vi "To Pythonic - Tuple.vi"(4 "Pythonic Values":string[](array[string])) -> (1 "Tuple":string)   [LabVIEW 2020, in "OPI.lvclass"]
doc: "Convert LabVIEW data into valid pythonic representation. \n\nThe input aray of strings should be valid pythonic values created with previous calls to To Pythonic converter."
uses:
  OPI.lvclass
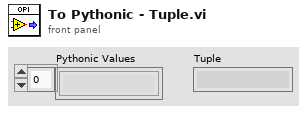
[diagram p1: front panel]
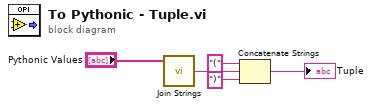
[diagram p0: block diagram]
diagram:
  n1 = call <vilib>:"Join Strings.vi"("Strings In"="Pythonic Values") -> ("String"=w1:string)  [unwired: 2 in]
  n2 = Concatenate Strings("(" ("string"), w1, ")" ("string")) -> (→"Tuple":string)
